vi "simple calculations.vi"() -> ()   [LabVIEW 2020]
panel:
  in  "Tab Control":enum32{"Page 1", "Page 2"}(tab)
  out "VNA App 2":cluster{"Frequency":dbl[], "S11_Imag":dbl[]}[](graph)
  out "VNA App 3":cluster{"Frequency":dbl[], "S11_Imag":dbl[]}[](graph)
  out "R140":cluster{"Frequency":dbl[], "S11_Imag":dbl[]}[](graph)
  out "VNA App":cluster{"Frequency":dbl[], "S21_Imag":dbl[]}[](graph)
  out "LV":cluster{"Frequency":dbl[], "S11_Imag":dbl[]}[](graph)
  out "VNA App 4":cluster{"Frequency":dbl[], "S11_Imag":dbl[]}[](graph)
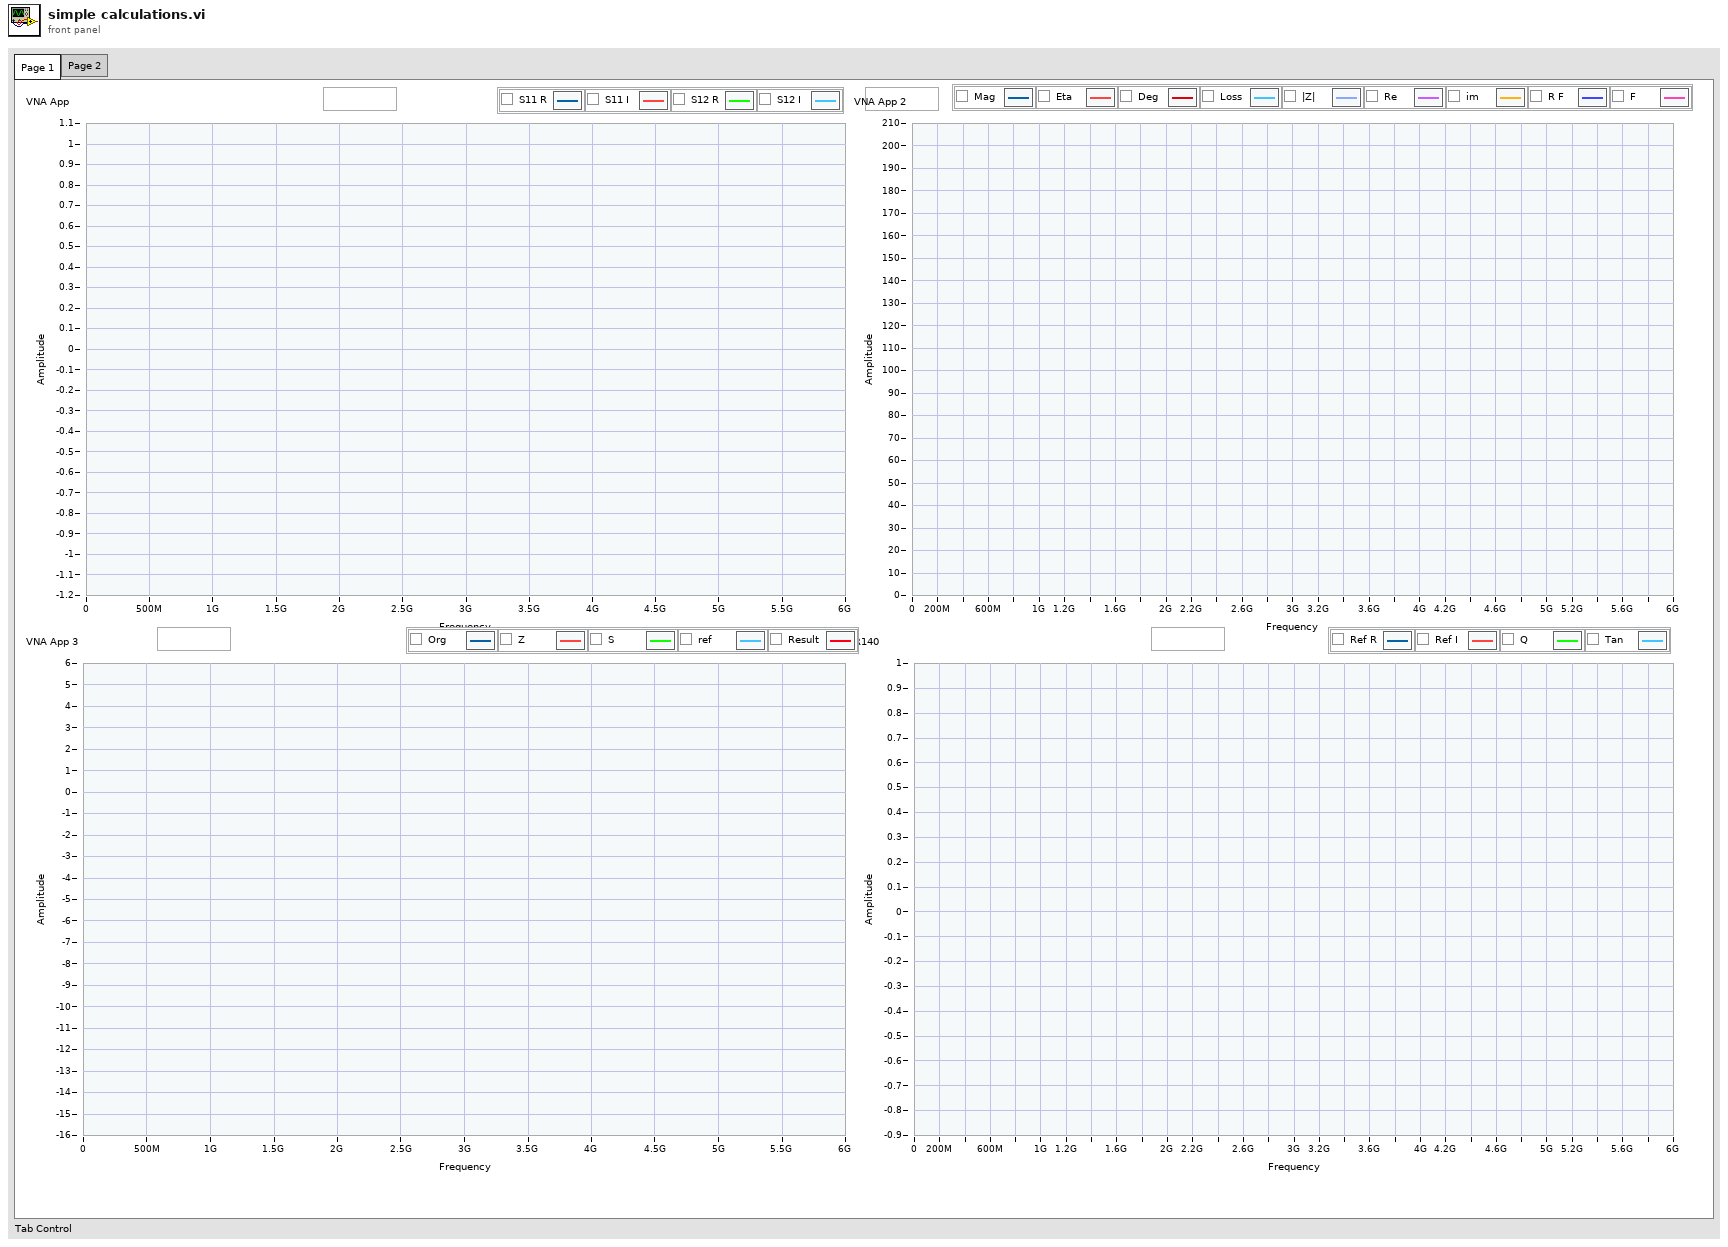
[diagram p1: front panel]
types:
  T1 = typedef "VFH-VNA_File_Handler.lvlib/VFH-file_cluster-Expensive.ctl" = cluster{"Frequency":dbl[], "Permativity'":dbl[], "Permativity''":dbl[], "Q [S/m]":dbl[], "Tan":dbl[], "Reflection R":dbl[], "Reflection I":dbl[]}
  T2 = typedef "VFH-VNA_File_Handler.lvlib/VFH-file_cluster-LabVIEWVNA.ctl" = cluster{"Frequency":dbl[], "S1_Real":dbl[], "S1_Imag":dbl[], "S11_Real":dbl[], "S11_Imag":dbl[], "S21_Real":dbl[], "S21_Imag":dbl[]}
  T3 = typedef "VFH-VNA_File_Handler.lvlib/VFH-file_cluster-NanoVNA.ctl" = cluster{"Frequency":dbl[], "S11_Real":dbl[], "S11_Imag":dbl[], "S21_Real":dbl[], "S21_Imag":dbl[], "S12_Real":dbl[], "S12_Imag":dbl[], "S22_Real":dbl[], "S22_Imag":dbl[]}
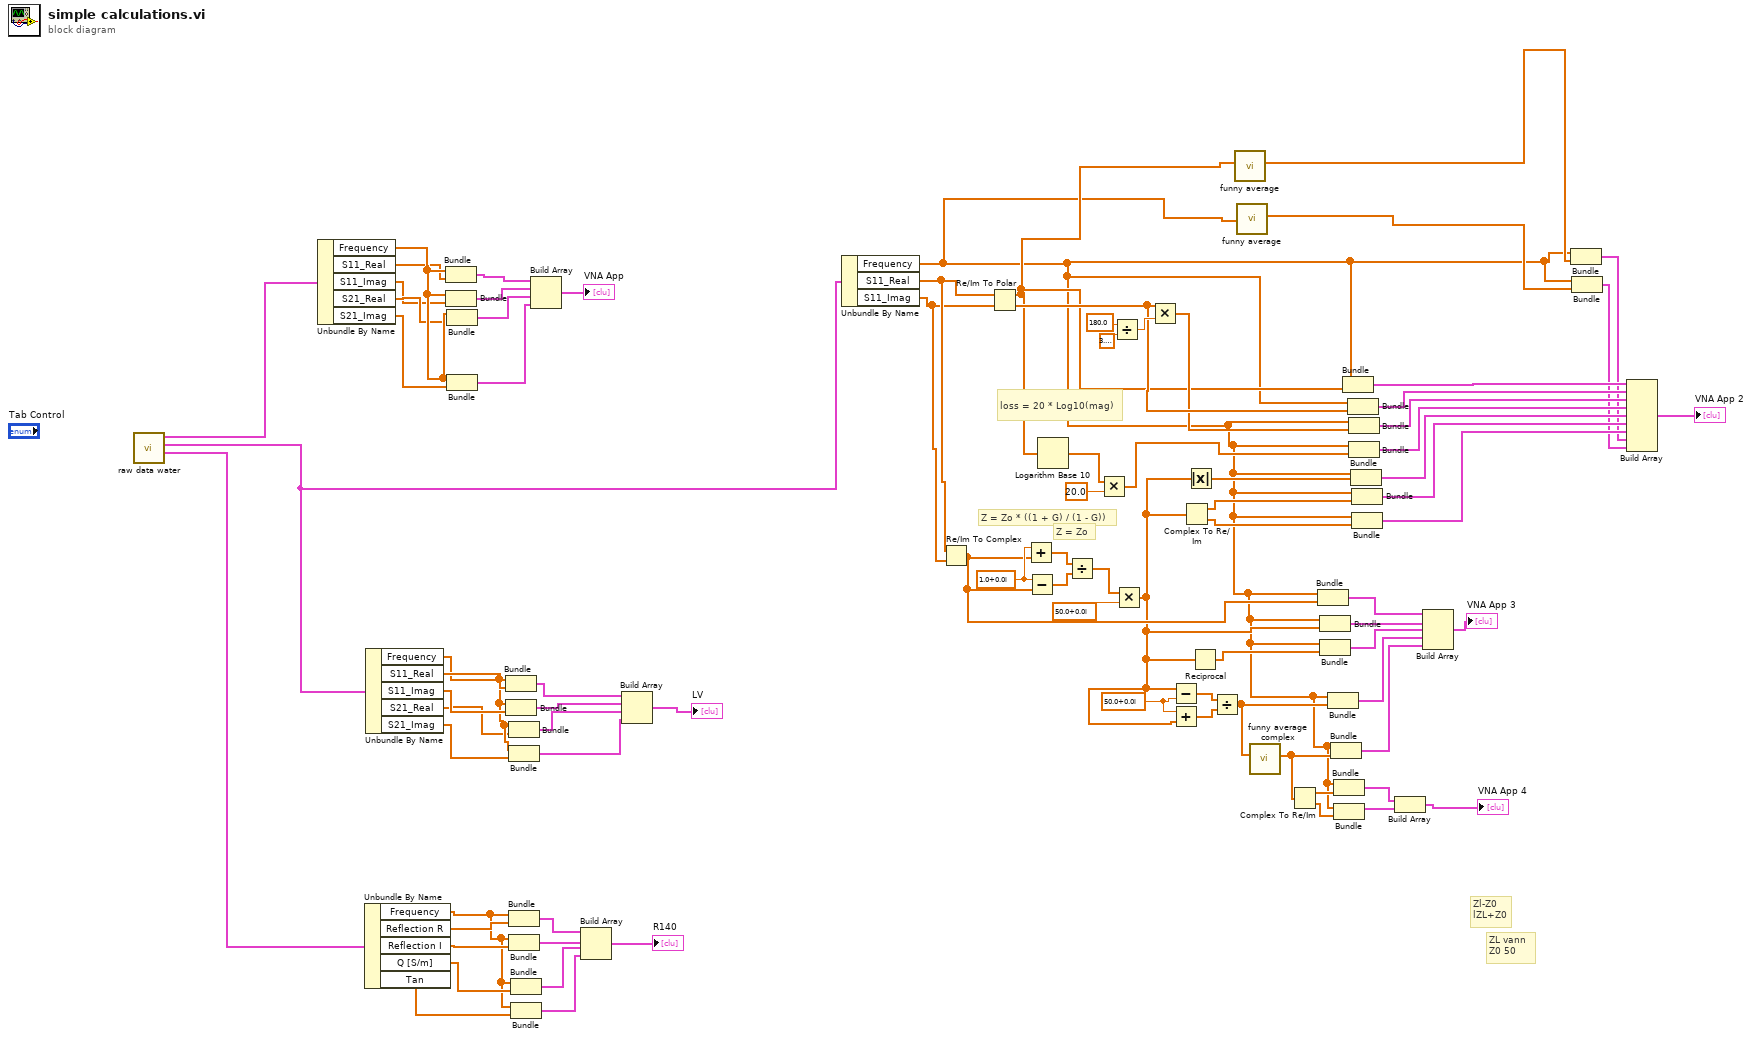
[diagram p0: block diagram]
diagram:
  w18 = cdb 50.0+0.0i ("y")
  w50 = cdb 1.0+0.0i ("x")
  # "ZL vann \nZ0 50"
  # "Zl-Z0\nlZL+Z0"
  # "Z = Zo"
  # "Z = Zo * ((1 + G) / (1 - G))"
  # "loss = 20 * Log10(mag)"
  n1 = call "raw data water.vi"() -> ("output R140"=w69:T1, "avg output LV"=w2:T2, "avg output NV"=w40:T3)  [unwired: 9 in]
  n2 = Unbundle By Name(w40) -> ("Frequency"=w82:dbl[], "S11_Real"=w15:dbl[], "S11_Imag"=w45:dbl[], "S21_Real"=w80:dbl[], "S21_Imag"=w81:dbl[])
  n3 = Unbundle By Name(w69) -> ("Frequency"=w59:dbl[], "Reflection R"=w70:dbl[], "Reflection I"=w71:dbl[], "Q [S/m]"=w61:dbl[], "Tan"=w60:dbl[])
  n4 = Unbundle By Name(w2) -> ("Frequency"=w66:dbl[], "S11_Real"=w75:dbl[], "S11_Imag"=w74:dbl[], "S21_Real"=w65:dbl[], "S21_Imag"=w64:dbl[])
  n5 = Bundle("Frequency"=w82, "S11_Real"=w15) -> (w78:cluster{"Frequency":dbl[], "S11_Real":dbl[]})  [unwired: 1 in]
  n6 = Bundle("Frequency"=w82, "S11_Imag"=w45) -> (w79:cluster{"Frequency":dbl[], "S11_Imag":dbl[]})  [unwired: 1 in]
  n7 = Bundle("Frequency"=w82, "S21_Real"=w80) -> (w83:cluster{"Frequency":dbl[], "S21_Real":dbl[]})  [unwired: 1 in]
  n8 = Bundle("Frequency"=w82, "S21_Imag"=w81) -> (w84:cluster{"Frequency":dbl[], "S21_Imag":dbl[]})  [unwired: 1 in]
  n9 = Bundle("Frequency"=w66, "S11_Real"=w75) -> (w76:cluster{"Frequency":dbl[], "S11_Real":dbl[]})  [unwired: 1 in]
  n10 = Bundle("Frequency"=w66, "S11_Imag"=w74) -> (w77:cluster{"Frequency":dbl[], "S11_Imag":dbl[]})  [unwired: 1 in]
  n11 = Bundle("Frequency"=w66, "S21_Real"=w65) -> (w63:cluster{"Frequency":dbl[], "S21_Real":dbl[]})  [unwired: 1 in]
  n12 = Bundle("Frequency"=w66, "S21_Imag"=w64) -> (w62:cluster{"Frequency":dbl[], "S21_Imag":dbl[]})  [unwired: 1 in]
  n13 = Bundle("Frequency"=w59, "Reflection R"=w70) -> (w72:cluster{"Frequency":dbl[], "Reflection R":dbl[]})  [unwired: 1 in]
  n14 = Bundle("Frequency"=w59, "Reflection I"=w71) -> (w73:cluster{"Frequency":dbl[], "Reflection I":dbl[]})  [unwired: 1 in]
  n15 = Bundle("Frequency"=w59, "Q [S/m]"=w61) -> (w58:cluster{"Frequency":dbl[], "Q [S/m]":dbl[]})  [unwired: 1 in]
  n16 = Bundle("Frequency"=w59, "Tan"=w60) -> (w57:cluster{"Frequency":dbl[], "Tan":dbl[]})  [unwired: 1 in]
  n17 = Build Array(w78, w79, w83, w84) -> (→"VNA App":cluster{"Frequency":dbl[], "S21_Imag":dbl[]}[])
  n18 = Build Array(w72, w73, w58, w57) -> (→"R140":cluster{"Frequency":dbl[], "Tan":dbl[]}[])
  n19 = Build Array(w76, w77, w63, w62) -> (→"LV":cluster{"Frequency":dbl[], "S21_Imag":dbl[]}[])
  n20 = Unbundle By Name(w2) -> ("Frequency"=w1:dbl[], "S11_Real"=w39:dbl[], "S11_Imag"=w22:dbl[])
  n21 = Re/Im To Complex(1:w22, 2:w39) -> (0:w16:cdb[])
  n22 = Re/Im To Polar(2:w22, 3:w39) -> (0:w37:dbl[], 1:w13:dbl[])
  n23 = Add(x=w50, y=w16) -> (x+y=w49:cdb[])
  n24 = Subtract(x=w50, y=w16) -> (x-y=w48:cdb[])
  n25 = Logarithm Base 10(1:w13) -> (0:w52:dbl[])
  n26 = Divide(x=w49, y=w48) -> (x/y=w47:cdb[])
  n27 = Multiply(x=w52, y=20.0) -> (x*y=w35:dbl[])
  n28 = Divide(x=180.0, y=3.141592653589793) -> (x/y=w53:dbl)
  n29 = Multiply(x=w47, y=cdb 50.0+0.0i) -> (x*y=w3:cdb[])
  n30 = Multiply(x=w37, y=w53) -> (x*y=w36:dbl[])
  n31 = Subtract(x=w3, y=w18) -> (x-y=w20:cdb[])
  n32 = Add(x=w18, y=w3) -> (x+y=w19:cdb[])
  n33 = Complex To Re/Im(x + iy=w3) -> (x=w33:dbl[], y=w32:dbl[])
  n34 = Absolute Value(x=w3) -> (abs(x)=w34:dbl[])
  n35 = Reciprocal(x=w3) -> (1/x=w38:cdb[])
  n36 = Divide(x=w20, y=w19) -> (x/y=w10:cdb[])
  n37 = call "funny average.vi"("in"=w13) -> ("Out"=w12:dbl[])  [unwired: 10 in]
  n38 = call "funny average.vi"("in"=w1) -> ("Out"=w14:dbl[])  [unwired: 10 in]
  n39 = call "funny average complex.vi"("in"=w10) -> ("Out"=w9:cdb[])  [unwired: 10 in]
  n40 = Complex To Re/Im(x + iy=w9) -> (x=w8:dbl[], y=w7:dbl[])
  n41 = Bundle("Frequency"=w1, w16) -> (w25:cluster{"Frequency":dbl[], cdb[]})  [unwired: 1 in]
  n42 = Bundle("Frequency"=w1, w3) -> (w26:cluster{"Frequency":dbl[], cdb[]})  [unwired: 1 in]
  n43 = Bundle("Frequency"=w1, w38) -> (w27:cluster{"Frequency":dbl[], cdb[]})  [unwired: 1 in]
  n44 = Bundle("Frequency"=w1, w10) -> (w17:cluster{"Frequency":dbl[], cdb[]})  [unwired: 1 in]
  n45 = Bundle("Frequency"=w1, "Out"=w9) -> (w11:cluster{"Frequency":dbl[], "Out":cdb[]})  [unwired: 1 in]
  n46 = Bundle("Frequency"=w1, w8) -> (w6:cluster{"Frequency":dbl[], dbl[]})  [unwired: 1 in]
  n47 = Bundle("Frequency"=w1, w7) -> (w5:cluster{"Frequency":dbl[], dbl[]})  [unwired: 1 in]
  n48 = Bundle("Frequency"=w1, w13) -> (w44:cluster{"Frequency":dbl[], dbl[]})  [unwired: 1 in]
  n49 = Bundle("Frequency"=w1, w37) -> (w43:cluster{"Frequency":dbl[], dbl[]})  [unwired: 1 in]
  n50 = Bundle("Frequency"=w1, w36) -> (w42:cluster{"Frequency":dbl[], dbl[]})  [unwired: 1 in]
  n51 = Bundle("Frequency"=w1, w35) -> (w41:cluster{"Frequency":dbl[], dbl[]})  [unwired: 1 in]
  n52 = Bundle("Frequency"=w1, w34) -> (w31:cluster{"Frequency":dbl[], dbl[]})  [unwired: 1 in]
  n53 = Bundle("Frequency"=w1, w33) -> (w30:cluster{"Frequency":dbl[], dbl[]})  [unwired: 1 in]
  n54 = Bundle("Frequency"=w1, w32) -> (w29:cluster{"Frequency":dbl[], dbl[]})  [unwired: 1 in]
  n55 = Build Array(w6, w5) -> (→"VNA App 4":cluster{"Frequency":dbl[], dbl[]}[])
  n56 = Build Array(w25, w26, w27, w17, w11) -> (→"VNA App 3":cluster{"Frequency":dbl[], "Out":cdb[]}[])
  n57 = Bundle("Frequency"=w1, "Out"=w12) -> (w23:cluster{"Frequency":dbl[], "Out":dbl[]})  [unwired: 1 in]
  n58 = Bundle("Frequency"=w1, "Out"=w14) -> (w21:cluster{"Frequency":dbl[], "Out":dbl[]})  [unwired: 1 in]
  n59 = Build Array(w44, w43, w42, w41, w31, w30, w29, w23, w21) -> (→"VNA App 2":cluster{"Frequency":dbl[], "Out":dbl[]}[])
